vi "总磷总氮通讯.vi"() -> ()   [LabVIEW 2016, in "斯坦道总磷总氮.lvlib"]
uses:
  <vilib>/Utility/config.llb/Write Key (Boolean).vi
  <vilib>/Utility/config.llb/Write Key (String).vi
  <vilib>/Plasmionique/MB Master/MB_Master/MB_Master.lvclass
  <vilib>/Utility/config.llb/NI_LVConfig.lvlib
  <vilib>/Plasmionique/MB Master/MB Master.lvlib
panel:
  out "序列号":string
  out "状态告警区":T1
  out "测量数据区":T2 {"单位" items=["ug/L", "mg/L", "ppm", "mg/m3", "cm", "ppb", "ug/m3", "%", "nmol/mol", "umol/mol", "MPN/L", "MPN/100ml", "ng/m3", "NTU", "无量纲", "ms/cm", "us/cm", "℃", "mV", "万个/L"]}
  out "status":bool
  out "关键参数区":T3
  in  "读关键参数区":bool
  in  "读状态告警区":bool
  in  "读测量数据区":bool
  in  "站号":u16(ring) items=["总磷"=1, "氨氮"=3]
  in  "停止":bool
  in  "启动":bool
  in  "控制命令":u16(ring) items=["启动测量"=1, "标样核查"=2, "零点核查"=3, "跨度核查"=4, "空白测试"=5, "平行样测试"=6, "加标回收"=7, "空白校准"=8, "标样校准"=9, "初始化（清洗）"=10, "停止测试"=11, "仪器重启"=12, "校时"=13, "模式设置"=14, "测量间隔设置"=15]
  in  "控制命令参数":u16[](array[numeric]) format="%04xH"
  in  "VISA Resource":refnum<visa-resource-name>
  in  "启用模块":bool
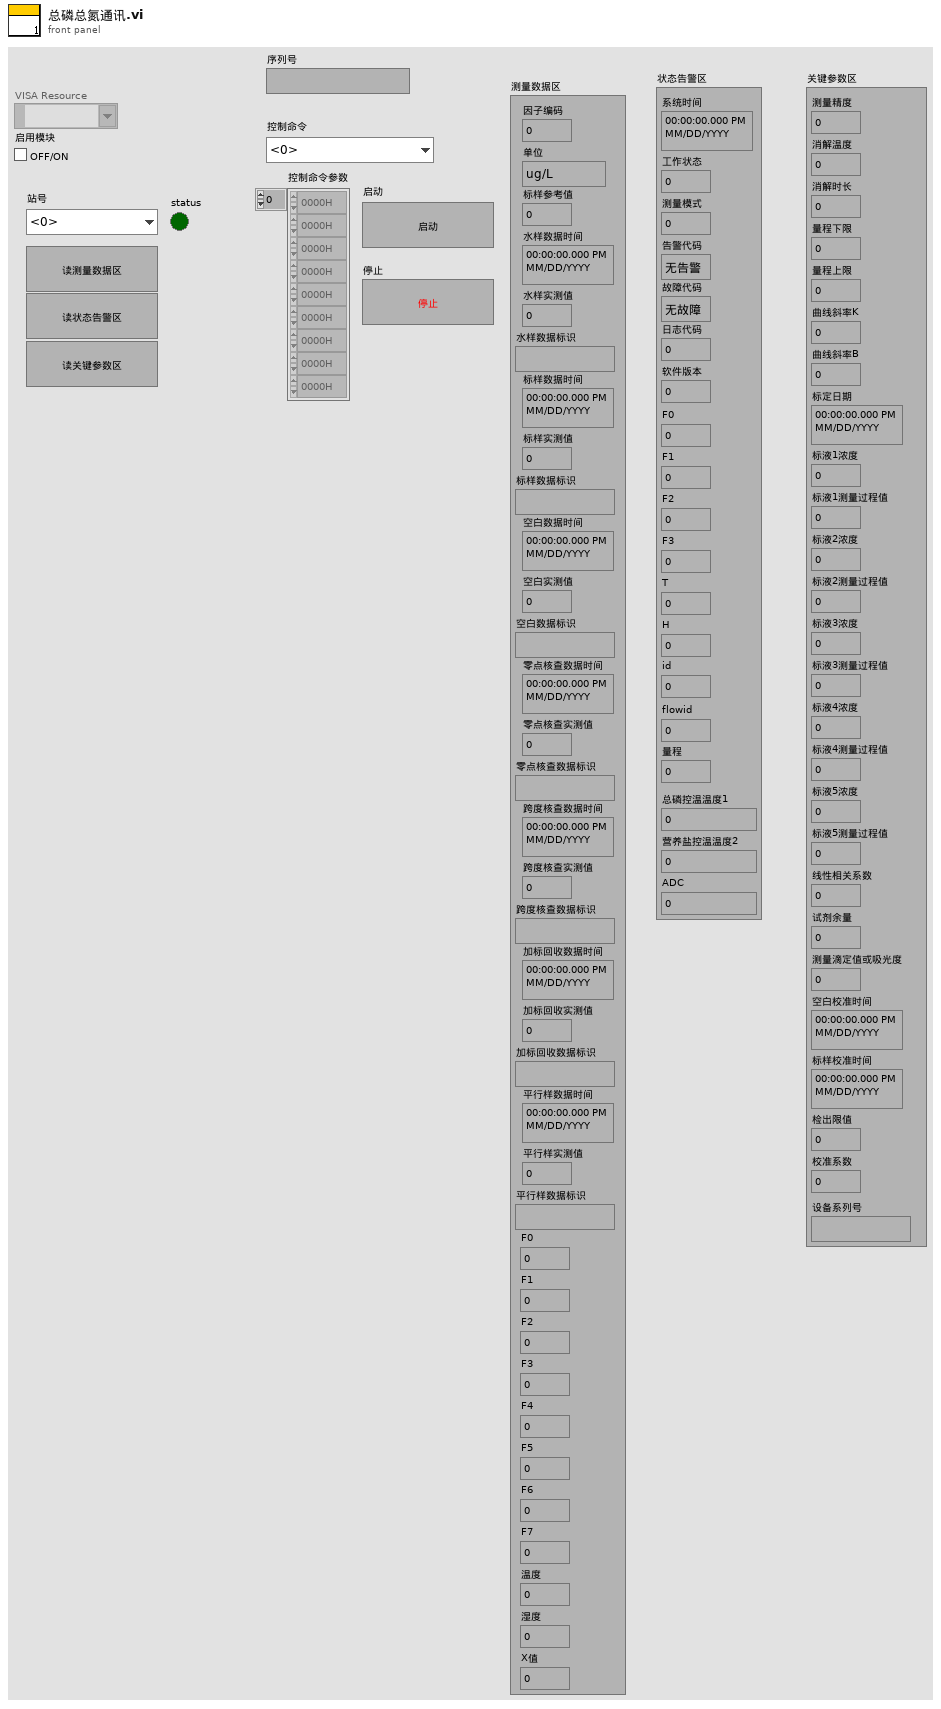
[diagram p1: front panel]
types:
  T1 = cluster{"系统时间":timestamp, "工作状态":u16, "测量模式":u16, "告警代码":enum16{"无告警", "缺试剂告警", "缺水样告警", "缺蒸馏水告警", "缺标液告警", "仪表漏液告警", "标定异常告警", "超量程告警", "加热异常", "低试剂预警", "超上限告警", "超下限告警", "仪表内部其他异常", "滴定异常告警", "电极异常告警", "量程切换告警", "参数设置告警", "PH电极电位异常", "电导率电极异常", "浊度光度异常", "溶解氧电极异常", "溶解氧光强异常", "温度异常告警", "PH异常告警", "溶解氧异常告警", "电导率异常告警", "浊度异常告警", "叶绿素异常告警", "藻密度异常告警", "蓝绿藻异常告警", "ORP异常告警", "氨氮异常告警", "清洁刷异常告警", "SD卡异常告警", "蓝牙异常告警", "Wifi异常告警", "流程异常告警"}, "故障代码":enum16{"无故障", "电机故障", "温度故障", "通讯故障", "滴定故障"}, "日志代码":u16, "软件版本":u16, "F0":sgl, "F1":sgl, "F2":sgl, "F3":sgl, "T":sgl, "H":sgl, "id":u16, "flowid":u16, "量程":u16, "总磷控温温度1":sgl, "营养盐控温温度2":sgl, "ADC":sgl}
  T2 = cluster{"因子编码":u32, "单位":u16, "标样参考值":sgl, "水样数据时间":timestamp, "水样实测值":sgl, "水样数据标识":string, "标样数据时间":timestamp, "标样实测值":sgl, "标样数据标识":string, "空白数据时间":timestamp, "空白实测值":sgl, "空白数据标识":string, "零点核查数据时间":timestamp, "零点核查实测值":sgl, "零点核查数据标识":string, "跨度核查数据时间":timestamp, "跨度核查实测值":sgl, "跨度核查数据标识":string, "加标回收数据时间":timestamp, "加标回收实测值":sgl, "加标回收数据标识":string, "平行样数据时间":timestamp, "平行样实测值":sgl, "平行样数据标识":string, "F0":sgl, "F1":sgl, "F2":sgl, "F3":sgl, "F4":sgl, "F5":sgl, "F6":sgl, "F7":sgl, "温度":sgl, "湿度":sgl, "X值":sgl}
  T3 = cluster{"测量精度":u16, "消解温度":u16, "消解时长":u16, "量程下限":sgl, "量程上限":sgl, "曲线斜率K":sgl, "曲线斜率B":sgl, "标定日期":timestamp, "标液1浓度":sgl, "标液1测量过程值":sgl, "标液2浓度":sgl, "标液2测量过程值":sgl, "标液3浓度":sgl, "标液3测量过程值":sgl, "标液4浓度":sgl, "标液4测量过程值":sgl, "标液5浓度":sgl, "标液5测量过程值":sgl, "线性相关系数":sgl, "试剂余量":u32, "测量滴定值或吸光度":sgl, "空白校准时间":timestamp, "标样校准时间":timestamp, "检出限值":sgl, "校准系数":sgl, "设备系列号":string}
  T4 = typedef "NI_LVConfig.lvlib/Config Data RefNum.ctl" = refnum<k1>
  T5 = enum8{"Enabled", "Disabled", "Disabled and Grayed Out"}
  T6 = cluster{"系统时间":timestamp, "工作状态":enum16{"空闲", "水样测试", "标样核查", "零点核查", "跨度核查", "空白测试", "平行样测试", "加标回收", "空白校准", "标样校准", "初始化（清洗）"}, "测量模式":enum16{"待机", "连续模式", "周期模式", "定点模式", "受控模式", "手动模式"}, "告警代码":enum16{"无告警", "缺试剂告警", "缺水样告警", "缺蒸馏水告警", "缺标液告警", "仪表漏液告警", "标定异常告警", "超量程告警", "加热异常", "低试剂预警", "超上限告警", "超下限告警", "仪表内部其他异常", "滴定异常告警", "电极异常告警", "量程切换告警", "参数设置告警", "PH电极电位异常", "电导率电极异常", "浊度光度异常", "溶解氧电极异常", "溶解氧光强异常", "温度异常告警", "PH异常告警", "溶解氧异常告警", "电导率异常告警", "浊度异常告警", "叶绿素异常告警", "藻密度异常告警", "蓝绿藻异常告警", "ORP异常告警", "氨氮异常告警", "清洁刷异常告警", "SD卡异常告警", "蓝牙异常告警", "Wifi异常告警", "流程异常告警"}, "故障代码":enum16{"无故障", "电机故障", "温度故障", "通讯故障", "滴定故障"}, "日志代码":u16, "软件版本":u16, "F0":sgl, "F1":sgl, "F2":sgl, "F3":sgl, "T":sgl, "H":sgl, "id":u16, "flowid":u16, "量程":u16, "总磷控温温度1":sgl, "营养盐控温温度2":sgl, "ADC":sgl}
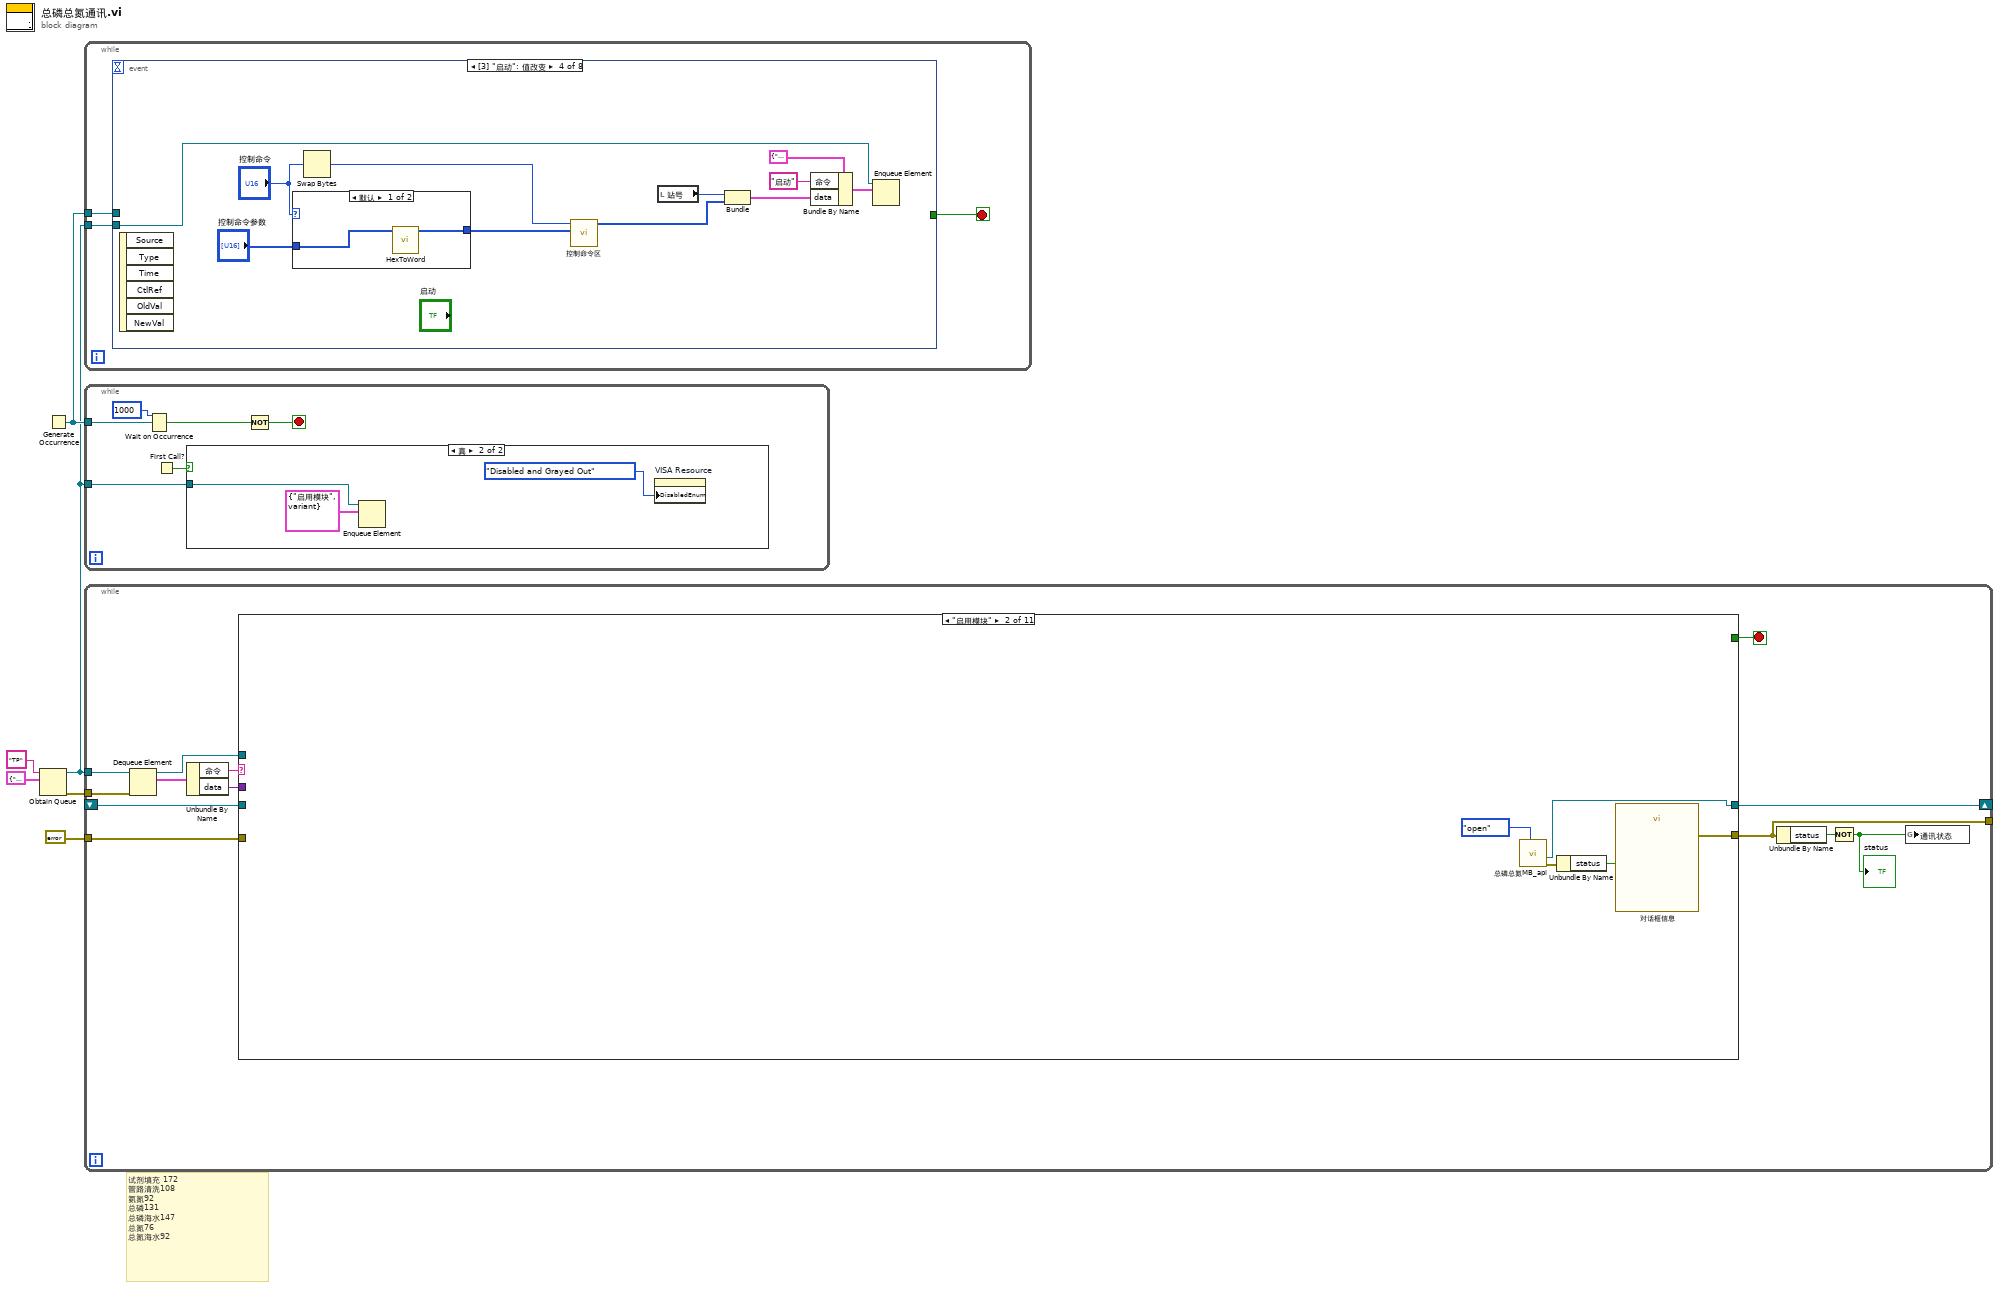
[diagram p0: block diagram]
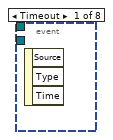
[diagram p3: hidden frame]
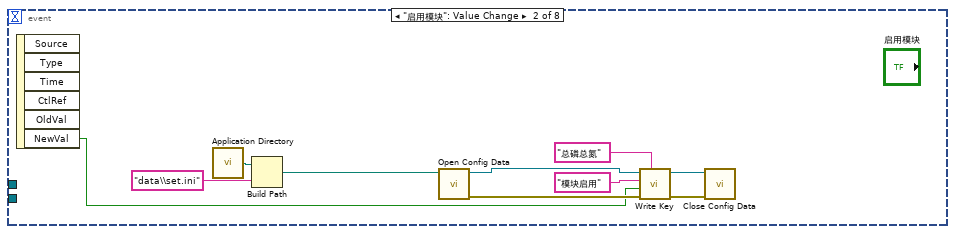
[diagram p4: hidden frame]
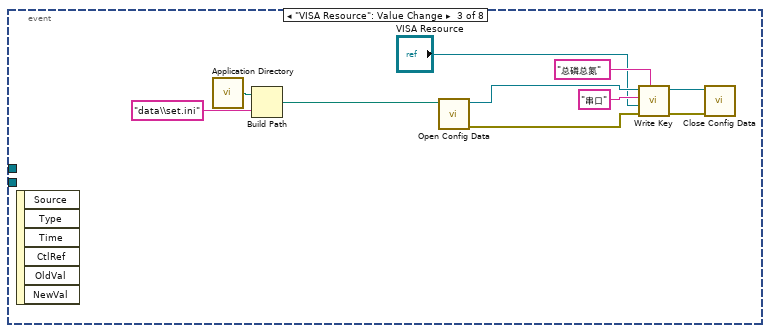
[diagram p5: hidden frame]
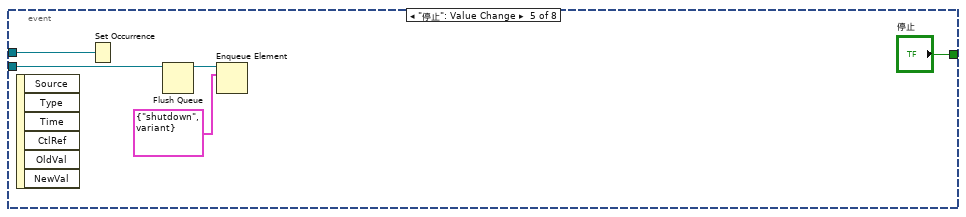
[diagram p7: hidden frame]
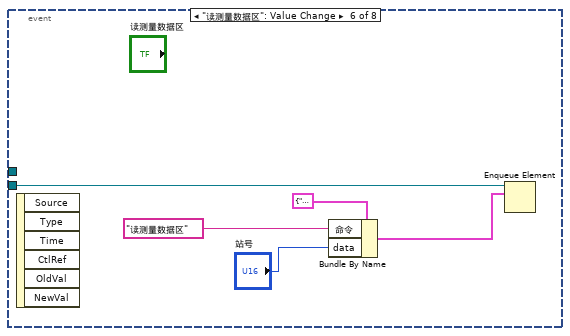
[diagram p8: hidden frame]
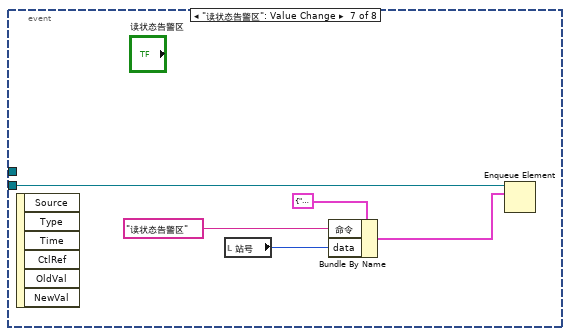
[diagram p9: hidden frame]
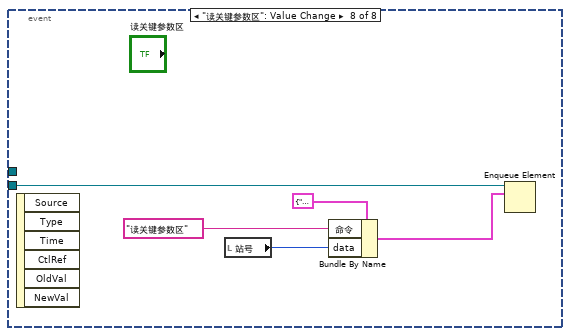
[diagram p10: hidden frame]
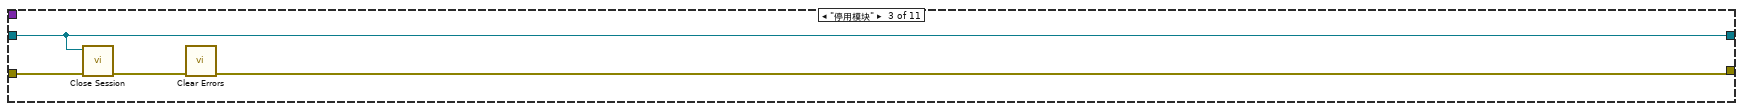
[diagram p12: hidden frame]
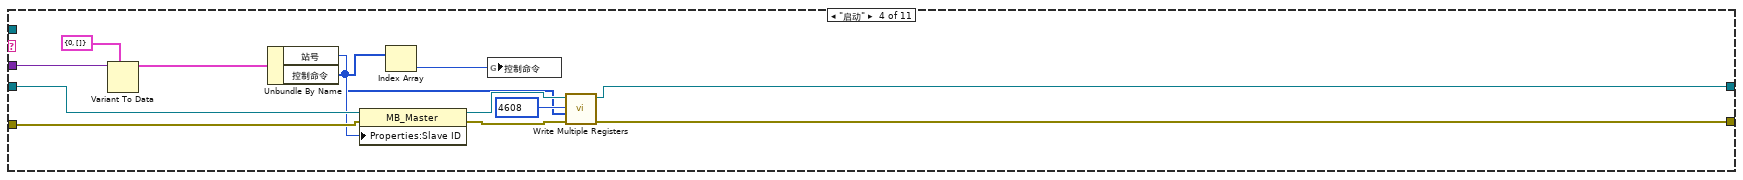
[diagram p13: hidden frame]
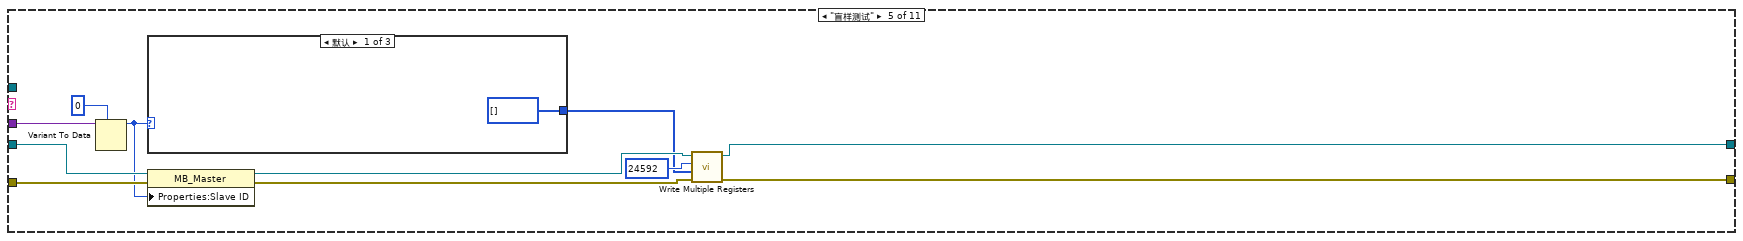
[diagram p14: hidden frame]
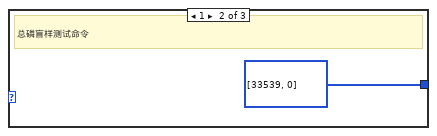
[diagram p15: hidden frame]
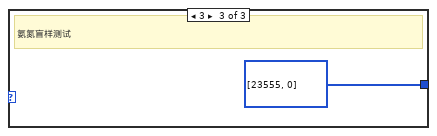
[diagram p16: hidden frame]
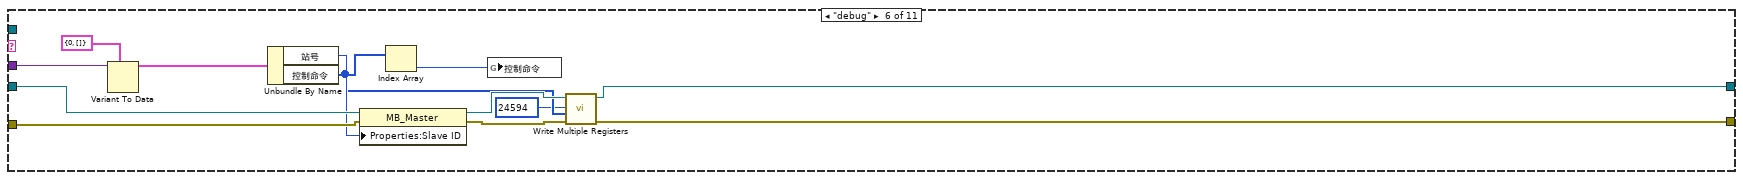
[diagram p17: hidden frame]
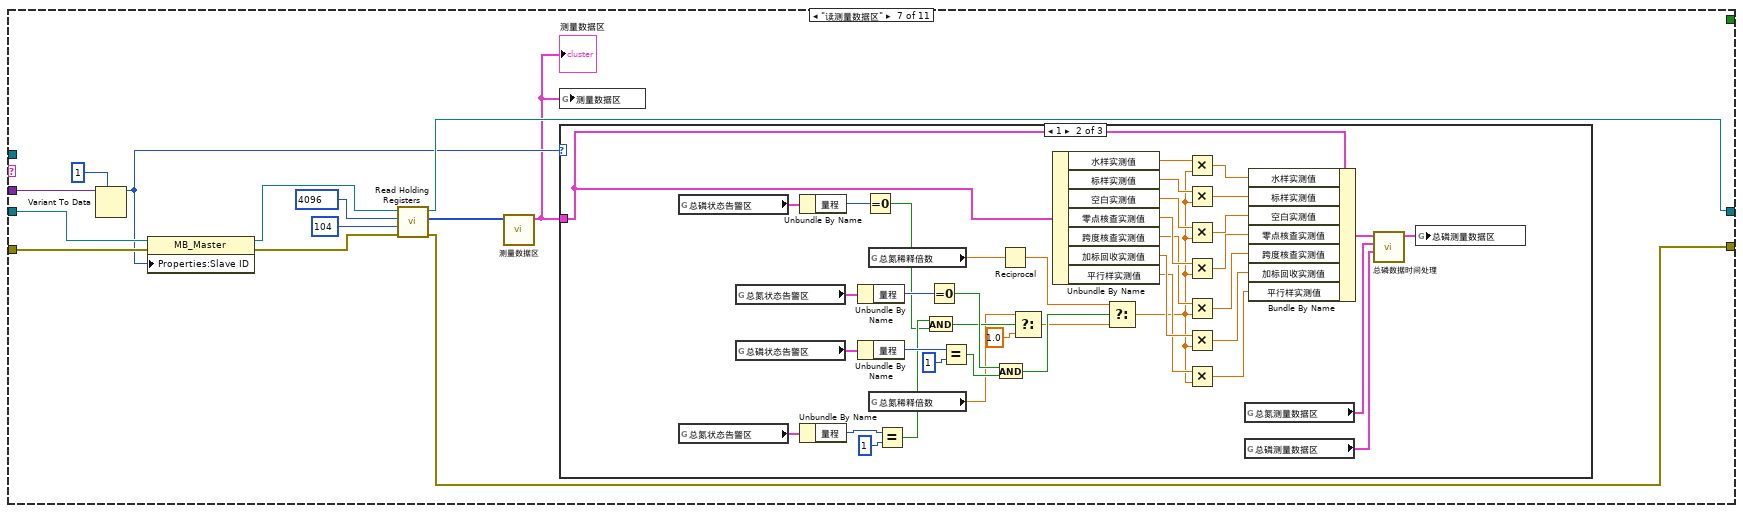
[diagram p18: hidden frame]
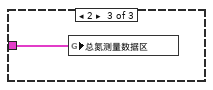
[diagram p20: hidden frame]
diagram:
  # "试剂填充 172 \n管路清洗108\n氨氮92\n总磷131\n总磷海水147\n总氮76\n总氮海水92"
  n1 = Obtain Queue(name (unnamed)="TP" ("名称（未命名）"), element data type=cluster{"命令":string, "data":variant} {"命令"="", "data"=variant}) -> (queue out=w1:refnum<queue>, error out=w4:errorcluster)  [unwired: 3 in, 1 out]
  n2 = Generate Occurrence() -> (w2:refnum<k4>)
  n3 = while {
    tunnel: w1 -> [w9]
    tunnel: w2 -> [w7]
    stop <- w8 stop-if-true
    n4 = event shown="[3] \"启动\": 值改变" {
      selector: _ -> [_ _ _ _ _ _ _ _]
      dyn-events: _ -> [_ _ _ _ _ _ _ _]
      timeout: _ -> [_ _ _ _ _ _ _ _]
      tunnel: w9 -> [_ _ _ w40 w47 w53 w58 w63]
      tunnel: [_ _ _ _ "停止" _ _ _] -> w8
      tunnel: w7 -> [_ _ _ _ w44 _ _ _]
      event Timeout {
        n5 = event-data() -> ()  [unwired: 1 in, 3 out]
      }
      event "启用模块": Value Change {
        n6 = event-data() -> ("NewVal"=w10:bool)  [unwired: 1 in, 5 out]
        n7 = call <vilib>:"Application Directory.vi"() -> ("Application Directory"=w12:path)
        n8 = Build Path(base path=w12, name or relative path="data\\set.ini" ("名称或相对路径")) -> (appended path=w13:path)
        n9 = call <vilib>:"Open Config Data.vi"("configuration file path"=w13) -> ("error out"=w19:errorcluster, "refnum"=w18:T4)  [unwired: 8 in, 1 out]
        n10 = call-poly <vilib>:"Write Key.vi"("section"="总磷总氮", "error in (no error)"=w19, "value"=w10, "key"="模块启用", "refnum"=w18) -> ("error out"=w15:errorcluster, "refnum out"=w11:T4)  [unwired: 4 in, 1 out]
        n11 = call <vilib>:"Close Config Data.vi"("error in (no error)"=w15, "refnum"=w11) -> ()  [unwired: 8 in, 2 out]
      }
      event "VISA Resource": Value Change {
        n12 = event-data() -> ()  [unwired: 1 in, 6 out]
        n13 = call <vilib>:"Application Directory.vi"() -> ("Application Directory"=w22:path)
        n14 = Build Path(base path=w22, name or relative path="data\\set.ini" ("名称或相对路径")) -> (appended path=w23:path)
        n15 = call <vilib>:"Open Config Data.vi"("configuration file path"=w23) -> ("error out"=w29:errorcluster, "refnum"=w28:T4)  [unwired: 8 in, 1 out]
        n16 = call-poly <vilib>:"Write Key.vi"("section"="总磷总氮", "error in (no error)"=w29, "value"="VISA Resource", "key"="串口", "refnum"=w28) -> ("error out"=w25:errorcluster, "refnum out"=w21:T4)  [unwired: 4 in, 1 out]
        n17 = call <vilib>:"Close Config Data.vi"("error in (no error)"=w25, "refnum"=w21) -> ()  [unwired: 8 in, 2 out]
      }
      event "启动": Value Change {
        n18 = event-data() -> ()  [unwired: 1 in, 6 out]
        n19 = case shown="默认" "控制命令" {
          tunnel: "控制命令参数" -> [w42 w43]
          tunnel: [w41 w43] -> w30
          frame Default {
            n20 = call "HexToWord.vi"("数组"=w42) -> ("WORD"=w41:u16[])  [unwired: 10 in]
          }
          frame 13 {
          }
        }
        n21 = Swap Bytes(anything="控制命令") -> (byte swapped=w33:u16)
        n22 = call "控制命令区.vi"("控制命令参数"=w30, "控制命令"=w33) -> ("控制命令"=w36:u16[])  [unwired: 9 in]
        n23 = local read "站号"() -> (w35:u16)
        n24 = Bundle("站号"=w35, "控制命令"=w36) -> (w34:cluster{"站号":u16, "控制命令":u16[]})  [unwired: 1 in]
        n25 = Bundle By Name(cluster=cluster{"命令":string, "data":variant} {"命令"="", "data"=variant} ("元素"), "命令"="启动", "data"=w34) -> (w38:cluster{"命令":string, "data":variant})
        n26 = Enqueue Element(queue=w40, element=w38) -> ()  [unwired: 2 in, 3 out]
      }
      event "停止": Value Change {
        n27 = event-data() -> ()  [unwired: 1 in, 6 out]
        n28 = Set Occurrence(w44) -> ()
        n29 = Flush Queue(queue=w47) -> (queue out=w46:refnum<queue>)  [unwired: 1 in, 2 out]
        n30 = Enqueue Element(queue=w46, element=cluster{"命令":string, "data":variant} {"命令"="shutdown", "data"=variant} ("元素")) -> ()  [unwired: 2 in, 3 out]
      }
      event "读测量数据区": Value Change {
        n31 = event-data() -> ()  [unwired: 1 in, 6 out]
        n32 = Bundle By Name(cluster=cluster{"命令":string, "data":variant} {"命令"="", "data"=variant} ("元素"), "命令"="读测量数据区", "data"="站号") -> (w51:cluster{"命令":string, "data":variant})
        n33 = Enqueue Element(queue=w53, element=w51) -> ()  [unwired: 2 in, 3 out]
      }
      event "读状态告警区": Value Change {
        n34 = event-data() -> ()  [unwired: 1 in, 6 out]
        n35 = local read "站号"() -> (w54:u16)
        n36 = Bundle By Name(cluster=cluster{"命令":string, "data":variant} {"命令"="", "data"=variant} ("元素"), "命令"="读状态告警区", "data"=w54) -> (w56:cluster{"命令":string, "data":variant})
        n37 = Enqueue Element(queue=w58, element=w56) -> ()  [unwired: 2 in, 3 out]
      }
      event "读关键参数区": Value Change {
        n38 = event-data() -> ()  [unwired: 1 in, 6 out]
        n39 = local read "站号"() -> (w59:u16)
        n40 = Bundle By Name(cluster=cluster{"命令":string, "data":variant} {"命令"="", "data"=variant} ("元素"), "命令"="读关键参数区", "data"=w59) -> (w61:cluster{"命令":string, "data":variant})
        n41 = Enqueue Element(queue=w63, element=w61) -> ()  [unwired: 2 in, 3 out]
      }
    }
  }
  n42 = while {
    tunnel: w2 -> [w69]
    tunnel: w1 -> [w65]
    stop <- w66 stop-if-true
    n43 = Wait on Occurrence(2:w69, 3:1000 ("毫秒超时(-1)")) -> (0:w67:bool)  [unwired: 1 in]
    n44 = First Call?() -> (First Call?: T/F=w64:bool)
    n45 = case shown="真" w64 {
      tunnel: w65 -> [_ w71]
      frame False {
      }
      frame True {
        n46 = Enqueue Element(queue=w71, element=cluster{"命令":string, "data":variant} {"命令"="启用模块", "data"=variant} ("元素")) -> ()  [unwired: 2 in, 3 out]
        n47 = property on="VISA Resource" class="VISAName"("DisabledEnum"=T5."Disabled and Grayed Out" ("禁用")) -> ()  [unwired: 2 in, 2 out]
      }
    }
    n48 = Not(x=w67) -> (.not. x?=w66:bool)
  }
  n49 = while {
    tunnel: w1 -> [w85]
    tunnel: w4 -> [w84]
    shift-right: [w82] -> _
    shift-left: _ -> [w81]
    tunnel: errorcluster {"status"=FALSE, "code"=0, "source"=""} ("error out") -> [w80]
    tunnel: [w75] -> _
    stop <- w83 stop-if-true
    n50 = Dequeue Element(queue=w85, error in (no error)=w84) -> (queue out=w76:refnum<queue>, element=w78:cluster{"命令":string, "data":variant})  [unwired: 1 in, 2 out]
    n51 = Unbundle By Name(w78) -> ("命令"=w79:string, "data"=w77:variant)
    n52 = case shown="\"启用模块\"" w79 {
      tunnel: w77 -> [_ _ _ w106 w117 w134 w144 w196 w212 w226 _]
      tunnel: w76 -> [_ _ _ _ _ _ _ _ _ _ w239]
      tunnel: [_ _ _ _ _ _ _ _ _ _ TRUE] -> w83
      tunnel: [w86 w88 w93 w109 w120 w136 w148 w205 w219 w233 w235] -> w82
      tunnel: [w87 w91 w94 w108 w119 w135 w149 w194 w220 w234 w236] -> w75
      tunnel: w81 -> [w86 _ w93 w105 w116 w133 w143 w199 w215 w229 w235]
      tunnel: w80 -> [w87 _ w96 w102 w113 w130 w141 w200 w216 w230 w237]
      frame Default {
      }
      frame "启用模块" {
        n53 = call "总磷总氮MB_api.vi"("STEP"=enum16{"open", "read", "write", "close"}."open") -> ("error out"=w89:errorcluster, "MB session out"=w88:refnum<class "MB_Master.lvclass">)  [unwired: 7 in, 2 out]
        n54 = Unbundle By Name(w89) -> ("status"=w92:bool)
        n55 = call "对话框信息"("Enable"=w92) -> ("error out"=w91:errorcluster)  [unwired: 9 in, 1 out]
      }
      frame "停用模块" {
        n56 = call-dynamic "Close Session.vi"("error in (no error)"=w96, "MB session in"=w93) -> ("error out"=w95:errorcluster)  [unwired: 9 in]
        n57 = call <vilib>:"Clear Errors.vi"("error in (no error)"=w95) -> ("error out"=w94:errorcluster)  [unwired: 5 in, 1 out]
      }
      frame "启动" {
        n58 = Variant To Data(type=cluster{"站号":u16, "控制命令":u16[]} {"站号"=0, "控制命令"=[]} ("输出簇"), Variant=w106) -> (data=w100:cluster{"站号":u16, "控制命令":u16[]})  [unwired: 1 in, 1 out]
        n59 = Unbundle By Name(w100) -> ("站号"=w99:u16, "控制命令"=w97:u16[])
        n60 = property class="MB_Master"(reference=w105, error in=w102, "Properties:Slave ID"=w99) -> (reference out=w104:refnum<class "MB_Master.lvclass">, error out=w103:errorcluster)
        n61 = Index Array(array=w97) -> (element=w98:u16)  [unwired: 1 in]
        n62 = global write "VAR总磷总氮全局变量.vi" "控制命令"(w98) -> ()
        n63 = call <vilib>:"Write Multiple Registers.vi"("error in (no error)"=w103, "values"=w97, "starting address"=u16 4608, "MB session in"=w104) -> ("error out"=w108:errorcluster, "MB session out"=w109:refnum<class "MB_Master.lvclass">)  [unwired: 6 in]
      }
      frame "盲样测试" {
        n64 = Variant To Data(type=0, Variant=w117) -> (data=w110:i32)  [unwired: 1 in, 1 out]
        n65 = case shown="默认" w110 {
          tunnel: [u16[] [] ("values") u16[] [33539, 0] ("values") u16[] [23555, 0] ("values")] -> w112
          frame Default {
          }
          frame 1 {
            # "总磷盲样测试命令"
          }
          frame 3 {
            # "氨氮盲样测试"
          }
        }
        n66 = property class="MB_Master"(reference=w116, error in=w113, "Properties:Slave ID"=w110) -> (reference out=w115:refnum<class "MB_Master.lvclass">, error out=w114:errorcluster)
        n67 = call <vilib>:"Write Multiple Registers.vi"("error in (no error)"=w114, "values"=w112, "starting address"=u16 24592, "MB session in"=w115) -> ("error out"=w119:errorcluster, "MB session out"=w120:refnum<class "MB_Master.lvclass">)  [unwired: 6 in]
      }
      frame "debug" {
        n68 = Variant To Data(type=cluster{"站号":u16, "控制命令":u16[]} {"站号"=0, "控制命令"=[]} ("输出簇"), Variant=w134) -> (data=w128:cluster{"站号":u16, "控制命令":u16[]})  [unwired: 1 in, 1 out]
        n69 = Unbundle By Name(w128) -> ("站号"=w127:u16, "控制命令"=w125:u16[])
        n70 = property class="MB_Master"(reference=w133, error in=w130, "Properties:Slave ID"=w127) -> (reference out=w132:refnum<class "MB_Master.lvclass">, error out=w131:errorcluster)
        n71 = Index Array(array=w125) -> (element=w126:u16)  [unwired: 1 in]
        n72 = global write "VAR总磷总氮全局变量.vi" "控制命令"(w126) -> ()
        n73 = call <vilib>:"Write Multiple Registers.vi"("error in (no error)"=w131, "values"=w125, "starting address"=u16 24594, "MB session in"=w132) -> ("error out"=w135:errorcluster, "MB session out"=w136:refnum<class "MB_Master.lvclass">)  [unwired: 6 in]
      }
      frame "读测量数据区" {
        n74 = Variant To Data(type=u8 1 ("Slave ID"), Variant=w144) -> (data=w138:u8)  [unwired: 1 in, 1 out]
        n75 = property class="MB_Master"(reference=w143, error in=w141, "Properties:Slave ID"=w138) -> (reference out=w142:refnum<class "MB_Master.lvclass">, error out=w140:errorcluster)
        n76 = call <vilib>:"Read Holding Registers.vi"("error in (no error)"=w140, "quantity"=u16 104, "starting address"=u16 4096, "MB session in"=w142) -> ("error out"=w149:errorcluster, "Registers"=w139:u16[], "MB session out"=w148:refnum<class "MB_Master.lvclass">)  [unwired: 5 in]
        n77 = call "测量数据区.vi"("数组"=w139) -> ("测量数据区"=w137:T2)  [unwired: 10 in]
        "测量数据区" <- w137
        n78 = global write "VAR总磷总氮全局变量.vi" "测量数据区"(w137) -> ()
        n79 = case shown="1" w138 {
          tunnel: w137 -> [_ w190 w191]
          frame 0, Default {
          }
          frame 1 {
            n80 = global read "VAR总磷总氮全局变量.vi" "总磷状态告警区"() -> (w159:T6)
            n81 = global read "VAR总磷总氮全局变量.vi" "总氮状态告警区"() -> (w158:T6)
            n82 = global read "VAR总磷总氮全局变量.vi" "总氮状态告警区"() -> (w170:T6)
            n83 = global read "VAR总磷总氮全局变量.vi" "总磷状态告警区"() -> (w169:T6)
            n84 = Unbundle By Name(w159) -> ("量程"=w155:u16)
            n85 = Unbundle By Name(w158) -> ("量程"=w157:u16)
            n86 = Unbundle By Name(w170) -> ("量程"=w168:u16)
            n87 = Unbundle By Name(w169) -> ("量程"=w167:u16)
            n88 = Equal To 0?(x=w155) -> (x = 0?=w160:bool)
            n89 = global read "总磷总氮断电保存全局变量.vi" "总氮稀释倍数"() -> (w150:dbl)
            n90 = global read "总磷总氮断电保存全局变量.vi" "总氮稀释倍数"() -> (w151:dbl)
            n91 = Equal?(x=w157, y=u16 1) -> (x = y?=w161:bool)
            n92 = And(x=w161, y=w160) -> (x .and. y?=w154:bool)
            n93 = Equal To 0?(x=w168) -> (x = 0?=w164:bool)
            n94 = Equal?(x=w167, y=u16 1) -> (x = y?=w165:bool)
            n95 = And(x=w164, y=w165) -> (x .and. y?=w163:bool)
            n96 = Reciprocal(x=w150) -> (1/x=w162:dbl)
            n97 = Select(t=w151, s=w154, f=1.0) -> (s? t:f=w152:dbl)
            n98 = Unbundle By Name(w190) -> ("水样实测值"=w189:sgl, "标样实测值"=w187:sgl, "空白实测值"=w185:sgl, "零点核查实测值"=w183:sgl, "跨度核查实测值"=w181:sgl, "加标回收实测值"=w179:sgl, "平行样实测值"=w177:sgl)
            n99 = Select(t=w162, s=w163, f=w152) -> (s? t:f=w175:dbl)
            n100 = Multiply(x=w189, y=w175) -> (x*y=w188:dbl)
            n101 = Multiply(x=w187, y=w175) -> (x*y=w186:dbl)
            n102 = Multiply(x=w185, y=w175) -> (x*y=w184:dbl)
            n103 = Multiply(x=w183, y=w175) -> (x*y=w182:dbl)
            n104 = Multiply(x=w181, y=w175) -> (x*y=w180:dbl)
            n105 = Multiply(x=w179, y=w175) -> (x*y=w178:dbl)
            n106 = Multiply(x=w177, y=w175) -> (x*y=w176:dbl)
            n107 = global read "VAR总磷总氮全局变量.vi" "总氮测量数据区"() -> (w173:T2)
            n108 = global read "VAR总磷总氮全局变量.vi" "总磷测量数据区"() -> (w171:T2)
            n109 = Bundle By Name(cluster=w190, "水样实测值"=w188, "标样实测值"=w186, "空白实测值"=w184, "零点核查实测值"=w182, "跨度核查实测值"=w180, "加标回收实测值"=w178, "平行样实测值"=w176) -> (w174:T2)
            n110 = call "总磷数据时间处理.vi"("总磷修正数据输入"=w171, "总氮原始数据"=w173, "总磷原始数据"=w174) -> ("总磷修正数据输出"=w172:T2)  [unwired: 8 in]
            n111 = global write "VAR总磷总氮全局变量.vi" "总磷测量数据区"(w172) -> ()
          }
          frame 2 {
            n112 = global write "VAR总磷总氮全局变量.vi" "总氮测量数据区"(w191) -> ()
          }
        }
      }
      frame "读状态告警区" {
        n113 = Variant To Data(type=u8 1 ("Slave ID"), Variant=w196) -> (data=w201:u8)  [unwired: 1 in, 1 out]
        n114 = property class="MB_Master"(reference=w199, error in=w200, "Properties:Slave ID"=w201) -> (reference out=w198:refnum<class "MB_Master.lvclass">, error out=w197:errorcluster)
        n115 = call <vilib>:"Read Holding Registers.vi"("error in (no error)"=w197, "quantity"=u16 29, "starting address"=u16 4224, "MB session in"=w198) -> ("error out"=w194:errorcluster, "Registers"=w195:u16[], "MB session out"=w205:refnum<class "MB_Master.lvclass">)  [unwired: 5 in]
        n116 = call "状态告警区.vi"("数组"=w195) -> ("状态告警区"=w192:T6)  [unwired: 10 in]
        "状态告警区" <- w192
        n117 = global write "VAR总磷总氮全局变量.vi" "状态告警区"(w192) -> ()
        n118 = Unbundle By Name(w192) -> ("id"=w193:u16)
        n119 = case shown="76" w193 {
          tunnel: w192 -> [_ w206 w207]
          frame 0, Default {
          }
          frame 131 {
            n120 = global write "VAR总磷总氮全局变量.vi" "总磷状态告警区"(w206) -> ()
          }
          frame 76 {
            n121 = global write "VAR总磷总氮全局变量.vi" "总氮状态告警区"(w207) -> ()
          }
        }
      }
      frame "读关键参数区" {
        n122 = Variant To Data(type=u8 1 ("Slave ID"), Variant=w212) -> (data=w210:u8)  [unwired: 1 in, 1 out]
        n123 = property class="MB_Master"(reference=w215, error in=w216, "Properties:Slave ID"=w210) -> (reference out=w214:refnum<class "MB_Master.lvclass">, error out=w213:errorcluster)
        n124 = call <vilib>:"Read Holding Registers.vi"("error in (no error)"=w213, "quantity"=u16 19, "starting address"=u16 4256, "MB session in"=w214) -> ("error out"=w220:errorcluster, "Registers"=w209:u16[], "MB session out"=w219:refnum<class "MB_Master.lvclass">)  [unwired: 5 in]
        n125 = call "关键参数区.vi"("数组"=w209) -> ("关键参数区"=w208:T3)  [unwired: 10 in]
        "关键参数区" <- w208
        n126 = global write "VAR总磷总氮全局变量.vi" "关键参数区"(w208) -> ()
      }
      frame "读序列号" {
        n127 = Variant To Data(type=u8 1 ("Slave ID"), Variant=w226) -> (data=w224:u8)  [unwired: 1 in, 1 out]
        n128 = property class="MB_Master"(reference=w229, error in=w230, "Properties:Slave ID"=w224) -> (reference out=w228:refnum<class "MB_Master.lvclass">, error out=w227:errorcluster)
        n129 = call <vilib>:"Read Holding Registers.vi"("error in (no error)"=w227, "quantity"=u16 6, "starting address"=u16 3, "MB session in"=w228) -> ("error out"=w234:errorcluster, "Registers"=w223:u16[], "MB session out"=w233:refnum<class "MB_Master.lvclass">)  [unwired: 5 in]
        n130 = call "HexToString.vi"("数组"=w223) -> ("STRING"=w222:string[])  [unwired: 10 in]
        n131 = Index Array(array=w222) -> (element=w221:string)  [unwired: 1 in]
        "序列号" <- w221
        n132 = global write "VAR总磷总氮全局变量.vi" "序列号"(w221) -> ()
      }
      frame "shutdown" {
        n133 = call-dynamic "Close Session.vi"("error in (no error)"=w237, "MB session in"=w235) -> ("error out"=w236:errorcluster)  [unwired: 9 in]
        n134 = Flush Queue(queue=w239) -> (queue out=w238:refnum<queue>)  [unwired: 1 in, 2 out]
        n135 = Release Queue(queue=w238) -> ()  [unwired: 2 in, 3 out]
      }
    }
    n136 = Unbundle By Name(w75) -> ("status"=w74:bool)
    n137 = Not(x=w74) -> (.not. x?=w73:bool)
    "status" <- w73
    n138 = global write "VAR总磷总氮全局变量.vi" "通讯状态"(w73) -> ()
  }
